vi "Sparse - Scale Problem Linear.vi"(8 "error in (no error)":errorcluster, 9 "Y Scaling limits":cluster{"Y lower":dbl, "Y upper":dbl}={"Y lower"=nan, "Y upper"=nan}, 10 "X Scaling limits":cluster{"X lower":dbl, "X upper":dbl}={"X lower"=0.0, "X upper"=1.0}, 11 "Problem":T1) -> (0 "error out":errorcluster, 1 "ymaxmin":cluster{"ymax":dbl, "ymin":dbl}, 2 "xmaxmin":cluster{"min":dbl, "max":dbl}[](array[cluster]), 3 "Scaled problem":T1)   [LabVIEW 2014]
doc: "Scales the problem similarly to the svm-scale tool bundled with libsvm.\nAlways use the output from this VI to scale the test set instead of scaling individually."
uses:
  LibSVM Sparse/Wrapper API/Controls/svm_problem.ctl
  LibSVM Sparse/Wrapper API/Controls/svm_node.ctl
  Controls/Statemachine_ScaleProblem.ctl
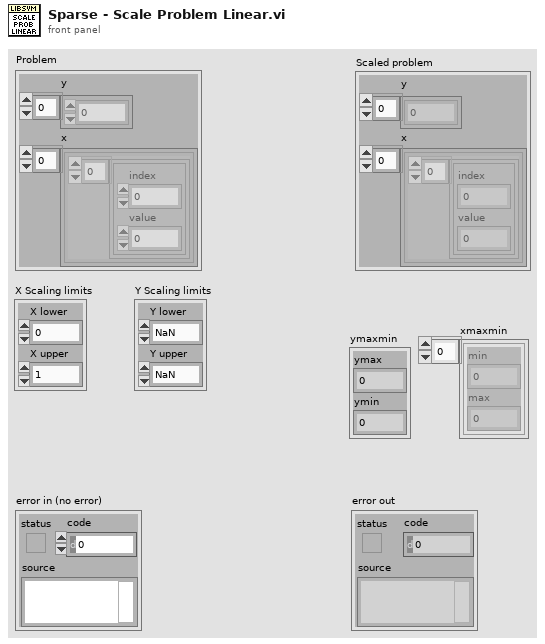
[diagram p1: front panel]
types:
  T1 = typedef "svm_problem.ctl" = cluster{"y":dbl[], "x":cluster{T2[]}[]}
  T2 = typedef "svm_node.ctl" = cluster{"index":i32, "value":dbl}
  T3 = typedef "Statemachine_ScaleProblem.ctl" = enum16{"Input verification: Limits", "Input verification: Ascending indices", "Find max/min index", "Find max/min features", "Scale", "Stop"}
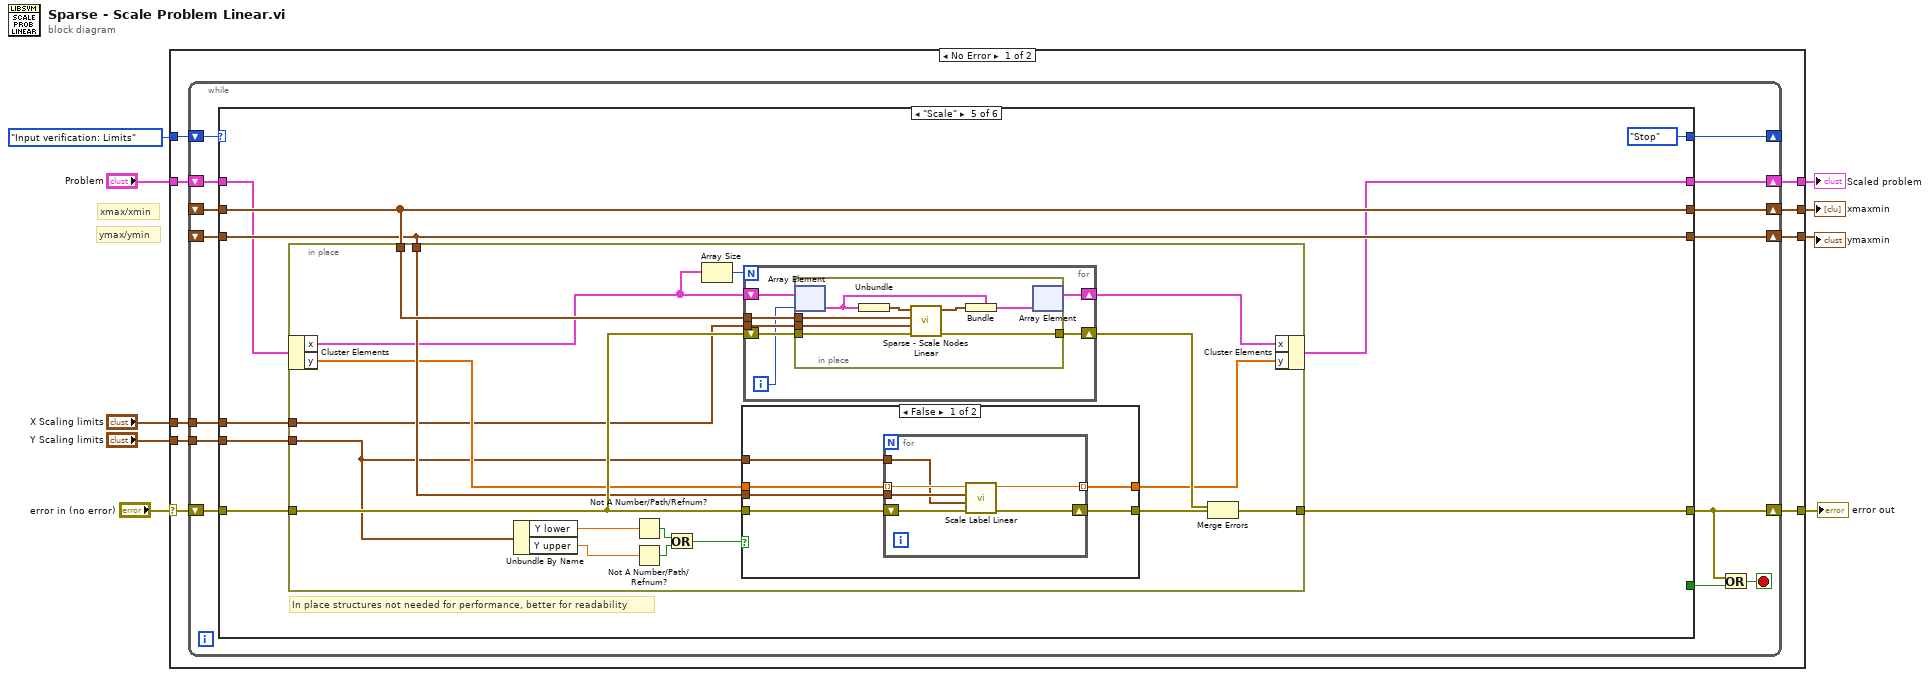
[diagram p0: block diagram]
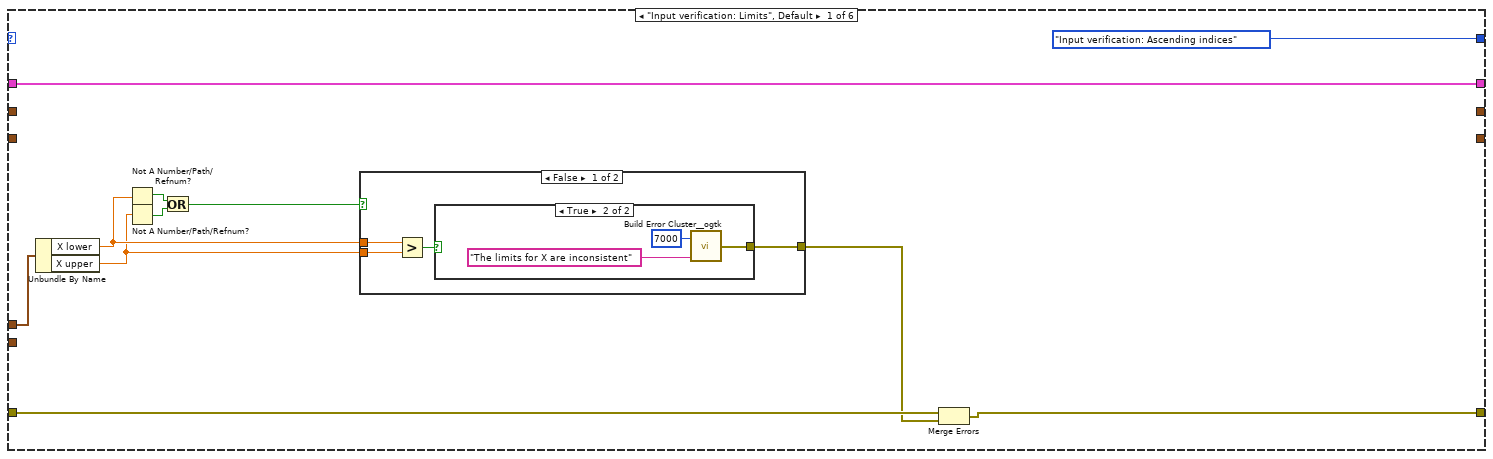
[diagram p2: hidden frame]
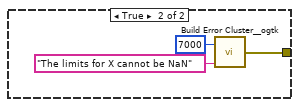
[diagram p4: hidden frame]
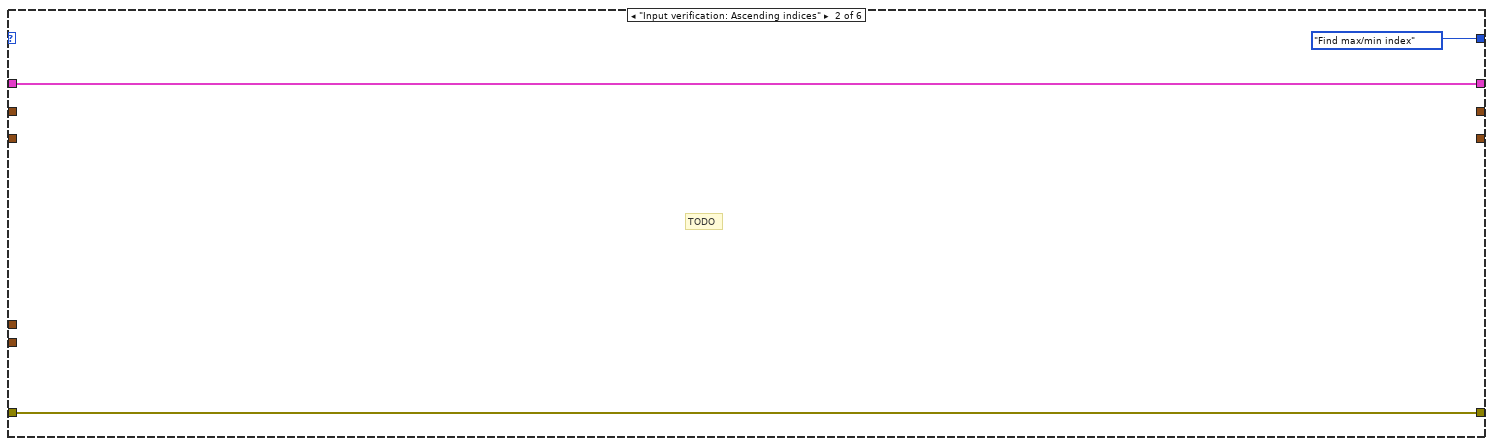
[diagram p5: hidden frame]
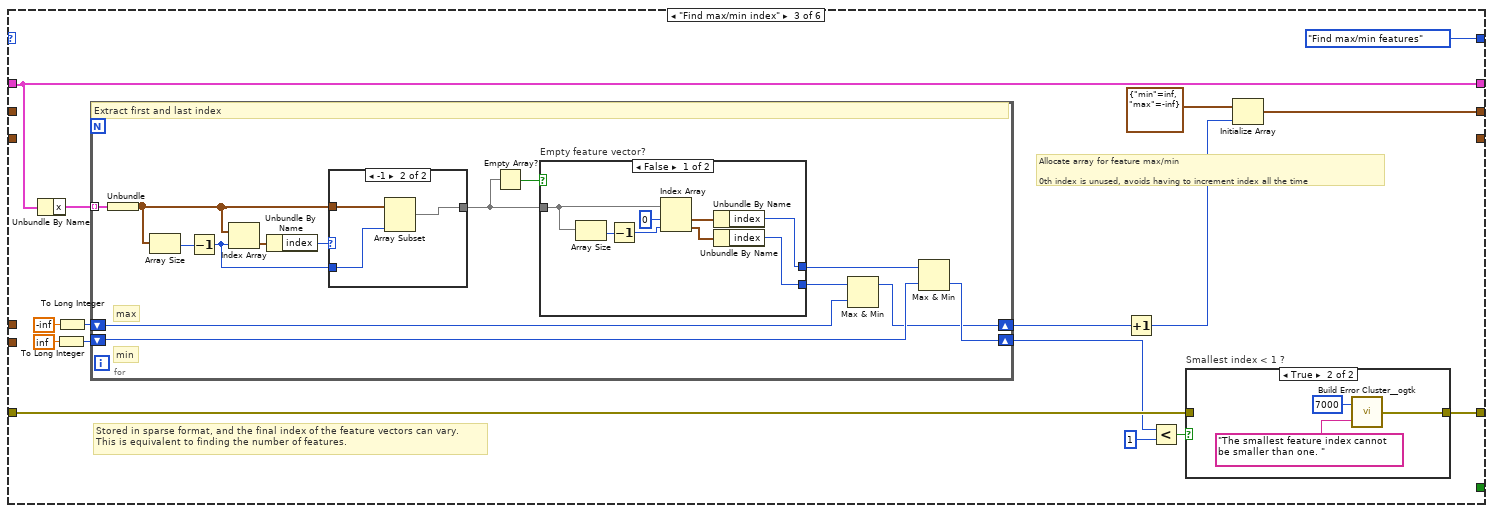
[diagram p6: hidden frame]
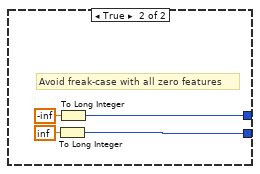
[diagram p9: hidden frame]
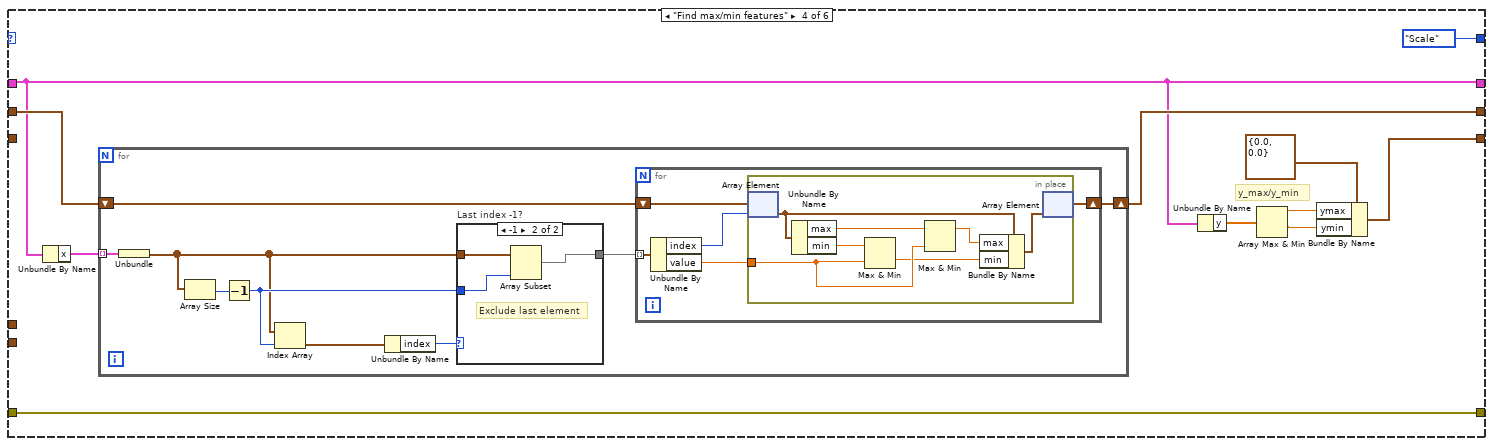
[diagram p10: hidden frame]
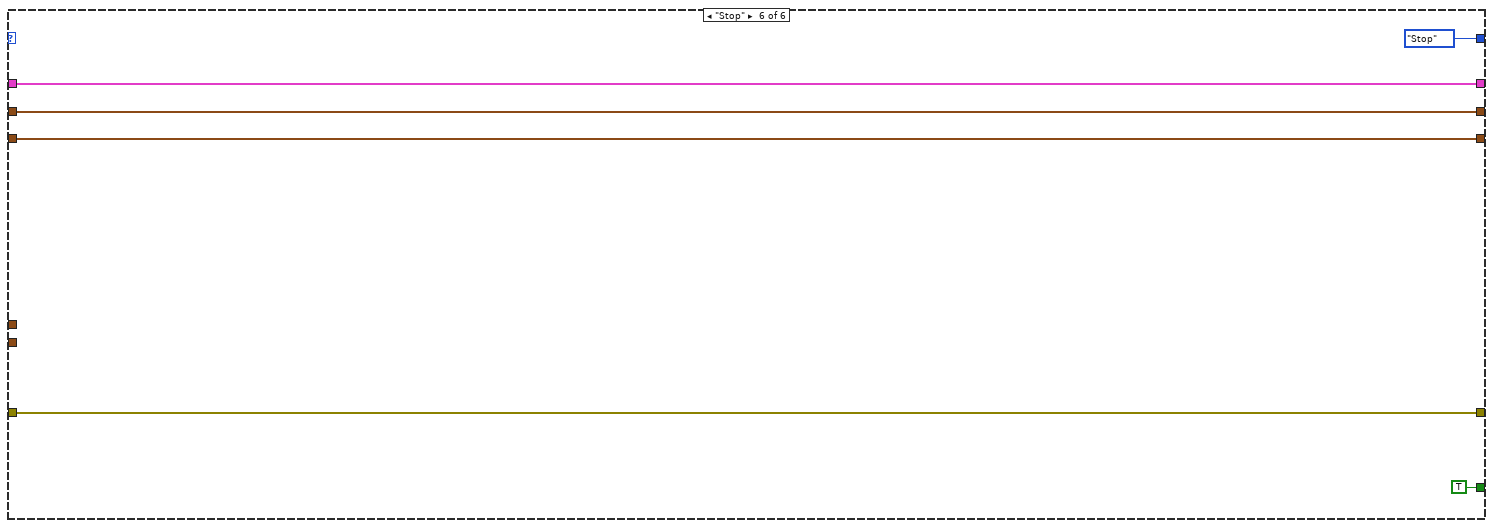
[diagram p13: hidden frame]
diagram:
  # "ymax/ymin"
  # "xmax/xmin"
  n1 = case shown="No Error" "error in (no error)" {
    selector: "error in (no error)" -> [w18 w205]
    tunnel: [w15 w205] -> w9
    tunnel: "Problem" -> [w11 _]
    tunnel: "X Scaling limits" -> [w16 _]
    tunnel: Statemachine_ScaleProblem."Input verification: Limits" ("Statemachine_ScaleProblem") -> [w17 _]
    tunnel: [w14 _] -> w3
    tunnel: [w13 _] -> w4
    tunnel: [w12 _] -> w2
    tunnel: "Y Scaling limits" -> [w10 _]
    frame No Error {
      n2 = while {
        shift-right: [w29] -> _
        shift-left: w17 -> [w32]
        tunnel: w16 -> [w31]
        shift-right: [w22] -> w15
        shift-left: w18 -> [w30]
        shift-right: [w28] -> w13
        shift-left: _ -> [w27]
        shift-right: [w26] -> w14
        shift-left: _ -> [w25]
        shift-right: [w24] -> w12
        shift-left: w11 -> [w23]
        tunnel: w10 -> [w19]
        stop <- w21 stop-if-true
        n3 = case shown="\"Scale\"" w32 {
          tunnel: w31 -> [w43 _ _ _ w150 _]
          tunnel: w30 -> [w37 w56 w64 w114 w149 w203]
          tunnel: [w35 w56 w65 w114 w148 w203] -> w22
          tunnel: [Statemachine_ScaleProblem."Input verification: Ascending indices" ("Statemachine_ScaleProblem") Statemachine_ScaleProblem."Find max/min index" ("Statemachine_ScaleProblem") Statemachine_ScaleProblem."Find max/min features" ("Statemachine_ScaleProblem") Statemachine_ScaleProblem."Scale" ("Statemachine_ScaleProblem") Statemachine_ScaleProblem."Stop" ("Statemachine_ScaleProblem") Statemachine_ScaleProblem."Stop" ("Statemachine_ScaleProblem")] -> w29
          tunnel: [_ _ w61 w115 w147 w202] -> w28
          tunnel: w27 -> [_ _ _ w116 w147 w202]
          tunnel: [_ _ _ w110 w146 w201] -> w26
          tunnel: w25 -> [_ _ _ _ w146 w201]
          tunnel: [w33 w54 w59 w108 w144 w200] -> w24
          tunnel: w23 -> [w33 w54 w59 w108 w145 w200]
          tunnel: [_ _ _ _ _ TRUE] -> w20
          tunnel: w19 -> [_ _ _ _ w143 _]
          frame "Input verification: Limits", Default {
            n4 = Unbundle By Name(w43) -> ("X lower"=w39:dbl, "X upper"=w38:dbl)
            n5 = Not A Number/Path/Refnum?(number/path/refnum=w39) -> (NaN/Path/Refnum?=w41:bool)
            n6 = Not A Number/Path/Refnum?(number/path/refnum=w38) -> (NaN/Path/Refnum?=w42:bool)
            n7 = Or(x=w41, y=w42) -> (x .or. y?=w40:bool)
            n8 = case shown="False" w40 {
              tunnel: w39 -> [w46 _]
              tunnel: w38 -> [w45 _]
              tunnel: [w44 w51] -> w36
              frame False {
                n9 = Greater?(x=w46, y=w45) -> (0:w47:bool)
                n10 = case shown="True" w47 {
                  tunnel: [_ w48] -> w44
                  frame False {
                  }
                  frame True {
                    n11 = call <userlib>:"Build Error Cluster__ogtk.vi"("String to Prepend to source (\"\")"="The limits for X are inconsistent" ("String to Prepend to source (\"\")"), "code"=7000) -> ("error out"=w48:errorcluster)
                  }
                }
              }
              frame True {
                n12 = call <userlib>:"Build Error Cluster__ogtk.vi"("String to Prepend to source (\"\")"="The limits for X cannot be NaN" ("String to Prepend to source (\"\")"), "code"=7000) -> ("error out"=w51:errorcluster)
              }
            }
            n13 = Merge Errors(w37, w36) -> (w35:errorcluster)
          }
          frame "Input verification: Ascending indices" {
            # "TODO"
          }
          frame "Find max/min index" {
            # "Allocate array for feature max/min\n\n0th index is unused, avoids having to increment index all the time"
            # "Stored in sparse format, and the final index of the feature vectors can vary.\nThis is equivalent to finding the number of features."
            n14 = Unbundle By Name(w59) -> ("x"=w72:cluster{T2[]}[])
            n15 = To Long Integer(number=inf) -> (32bit integer=w70:i32)
            n16 = To Long Integer(number=-inf) -> (32bit integer=w68:i32)
            n17 = for {
              tunnel: w72 -> [w90] mode=indexing
              shift-right: [w84] -> w58
              shift-left: w68 -> [w88]
              shift-right: [w85] -> w62
              shift-left: w70 -> [w86]
              # "min"
              # "max"
              # "Extract first and last index"
              n18 = Unbundle(w90) -> (w79:T2[])
              n19 = Array Size(array=w79) -> (size(s)=w82:i32)
              n20 = Decrement(x=w82) -> (x-1=w78:i32)
              n21 = Index Array(array=w79, index=w78) -> (element=w81:T2)
              n22 = Unbundle By Name(w81) -> ("index"=w80:i32)
              n23 = case shown="-1" w80 {
                tunnel: w79 -> [w91 w94]
                tunnel: w78 -> [_ w93]
                tunnel: [w91 w92] -> w77
                frame Default {
                }
                frame -1 {
                  n24 = Array Subset(array=w94, length=w93) -> (w92:T2[])  [unwired: 1 in]
                }
              }
              n25 = Empty Array?(array=w77) -> (empty?=w89:bool)
              n26 = case "Empty feature vector?" shown="False" w89 {
                tunnel: [w95 w103] -> w83
                tunnel: [w100 w104] -> w87
                tunnel: w77 -> [w98 _]
                frame False {
                  n27 = Array Size(array=w98) -> (size(s)=w97:i32)
                  n28 = Decrement(x=w97) -> (x-1=w96:i32)
                  n29 = Index Array(array=w98, index #1=0 ("index"), index #2=w96) -> (element #1=w101:T2, element #2=w99:T2)
                  n30 = Unbundle By Name(w101) -> ("index"=w100:i32)
                  n31 = Unbundle By Name(w99) -> ("index"=w95:i32)
                }
                frame True {
                  # "Avoid freak-case with all zero features"
                  n32 = To Long Integer(number=inf) -> (32bit integer=w103:i32)
                  n33 = To Long Integer(number=-inf) -> (32bit integer=w104:i32)
                }
              }
              n34 = Max & Min(x=w83, y=w88) -> (max(x,y)=w84:i32)  [unwired: 1 out]
              n35 = Max & Min(x=w87, y=w86) -> (min(x,y)=w85:i32)  [unwired: 1 out]
            }
            n36 = Increment(x=w58) -> (x+1=w57:i32)
            n37 = Less?(x=w62, y=1) -> (x < y?=w66:bool)
            n38 = case "Smallest index < 1 ?" shown="True" w66 {
              tunnel: [w73 w76] -> w65
              tunnel: w64 -> [w73 _]
              frame False {
              }
              frame True {
                n39 = call <userlib>:"Build Error Cluster__ogtk.vi"("String to Prepend to source (\"\")"="The smallest feature index cannot be smaller than one. " ("String to Prepend to source (\"\")"), "code"=7000) -> ("error out"=w76:errorcluster)
              }
            }
            n40 = Initialize Array(cluster{"min":dbl, "max":dbl} {"min"=inf, "max"=-inf}, w57) -> (w61:cluster{"min":dbl, "max":dbl}[])
          }
          frame "Find max/min features" {
            # "y_max/y_min"
            n41 = Unbundle By Name(w108) -> ("x"=w117:cluster{T2[]}[])
            n42 = for {
              tunnel: w117 -> [w126] mode=indexing
              shift-right: [w119] -> w115
              shift-left: w116 -> [w125]
              n43 = Unbundle(w126) -> (w118:T2[])
              n44 = Array Size(array=w118) -> (size(s)=w124:i32)
              n45 = Decrement(x=w124) -> (x-1=w121:i32)
              n46 = Index Array(array=w118, index=w121) -> (element=w123:T2)
              n47 = Unbundle By Name(w123) -> ("index"=w122:i32)
              n48 = case "Last index -1?" shown="-1" w122 {
                tunnel: w118 -> [w127 w130]
                tunnel: w121 -> [_ w129]
                tunnel: [w127 w128] -> w120
                frame Default {
                }
                frame -1 {
                  # "Exclude last element"
                  n49 = Array Subset(array=w130, length=w129) -> (w128:T2[])  [unwired: 1 in]
                }
              }
              n50 = for {
                tunnel: w120 -> [w135] mode=indexing
                shift-right: [w131] -> w119
                shift-left: w125 -> [w134]
                n51 = Unbundle By Name(w135) -> ("index"=w133:i32, "value"=w132:dbl)
                n52 = in-place {
                  in-place-border: w132 -> [w140]
                  n53 = in-place-array #1(w134, w133) -> (w139:cluster{"min":dbl, "max":dbl})
                  n54 = Unbundle By Name(w139) -> ("max"=w141:dbl, "min"=w142:dbl)
                  n55 = Max & Min(x=w142, y=w140) -> (min(x,y)=w137:dbl)  [unwired: 1 out]
                  n56 = Max & Min(x=w141, y=w140) -> (max(x,y)=w136:dbl)  [unwired: 1 out]
                  n57 = Bundle By Name(cluster=w139, "max"=w136, "min"=w137) -> (w138:cluster{"min":dbl, "max":dbl})
                  n58 = in-place-array #1(w138) -> (w131:cluster{"min":dbl, "max":dbl}[])  [unwired: 1 out]
                }
              }
            }
            n59 = Unbundle By Name(w108) -> ("y"=w107:dbl[])
            n60 = Array Max & Min(array=w107) -> (max value=w112:dbl, min value=w111:dbl)  [unwired: 2 out]
            n61 = Bundle By Name(cluster=cluster{"ymax":dbl, "ymin":dbl} {"ymax"=0.0, "ymin"=0.0}, "ymax"=w112, "ymin"=w111) -> (w110:cluster{"ymax":dbl, "ymin":dbl})
          }
          frame "Scale" {
            # "In place structures not needed for performance, better for readability"
            n62 = in-place {
              in-place-border: w150 -> [w153]
              in-place-border: w149 -> [w169]
              in-place-border: [w168] -> w148
              in-place-border: w147 -> [w162]
              in-place-border: w146 -> [w161]
              in-place-border: w143 -> [w152]
              n63 = in-place-cluster #2(w145) -> ("x"=w157:cluster{T2[]}[], "y"=w160:dbl[])
              n64 = Unbundle By Name(w152) -> ("Y lower"=w155:dbl, "Y upper"=w154:dbl)
              n65 = Not A Number/Path/Refnum?(number/path/refnum=w155) -> (NaN/Path/Refnum?=w165:bool)
              n66 = Not A Number/Path/Refnum?(number/path/refnum=w154) -> (NaN/Path/Refnum?=w164:bool)
              n67 = Or(x=w165, y=w164) -> (x .or. y?=w163:bool)
              n68 = Array Size(array=w157) -> (size(s)=w158:i32)
              n69 = case shown="False" w163 {
                tunnel: w169 -> [w175 w182]
                tunnel: w160 -> [w174 w183]
                tunnel: w161 -> [w173 _]
                tunnel: [w172 w182] -> w167
                tunnel: [w171 w183] -> w159
                tunnel: w152 -> [w170 _]
                frame False {
                  n70 = for {
                    shift-right: [w180] -> w172
                    shift-left: w175 -> [w181]
                    tunnel: w174 -> [w179] mode=indexing
                    tunnel: w170 -> [w176]
                    tunnel: w173 -> [w178]
                    tunnel: [w177] -> w171 mode=indexing
                    n71 = call "Scale Label Linear.vi"("error in (no error)"=w181, "Scaling limits"=w176, "ymaxmin"=w178, "y"=w179) -> ("error out"=w180:errorcluster, "y scaled"=w177:dbl)  [unwired: 6 in]
                  }
                }
                frame True {
                  # "NaN y limit - do not perform scaling"
                }
              }
              n72 = for {
                N: w158 -> [_]
                tunnel: w162 -> [w189]
                shift-right: [w188] -> w166
                shift-left: w169 -> [w190]
                tunnel: w153 -> [w187]
                shift-right: [w184] -> w156
                shift-left: w157 -> [w186]
                i -> [w185]
                n73 = in-place {
                  in-place-border: w190 -> [w197]
                  in-place-border: w189 -> [w198]
                  in-place-border: [w196] -> w188
                  in-place-border: w187 -> [w191]
                  n74 = in-place-array #3(w186, w185) -> (w192:cluster{T2[]})
                  n75 = Unbundle(w192) -> (w195:T2[])
                  n76 = call "Sparse - Scale Nodes Linear.vi"("error in (no error)"=w197, "Scaling limits"=w191, "xmaxmin"=w198, "x"=w195) -> ("error out"=w196:errorcluster, "x scaled"=w194:T2[])  [unwired: 6 in]
                  n77 = Bundle(cluster=w192, w194) -> (w193:cluster{T2[]})
                  n78 = in-place-array #3(w193) -> (w184:cluster{T2[]}[])  [unwired: 1 out]
                }
              }
              n79 = Merge Errors(w166, w167) -> (w168:errorcluster)
              n80 = in-place-cluster #2("x"=w156, "y"=w159) -> (w144:T1)
            }
          }
          frame "Stop" {
          }
        }
        n81 = Or(x=w22, y=w20) -> (x .or. y?=w21:bool)
      }
    }
    frame Error {
    }
  }
  "error out" <- w9
  "xmaxmin" <- w4
  "ymaxmin" <- w3
  "Scaled problem" <- w2
